vi "RDV-simpleGUI.vi"() -> ()   [LabVIEW 2020, in "RDV-Reflection_Data_viewer.lvclass"]
uses:
  RDV-Reflection_Data_viewer.lvclass
  RDV-PRELAUNCH_DATA.ctl
  RDV-XY_GRAPH_REFS.ctl
  RDV-GUI_REFS.ctl
panel:
  in  "Toggle Plot":bool
  in  "Stop":bool
  out "error out":errorcluster
  out "Permittivity Imag":T1(graph)
  out "Permittivity Real":T1(graph)
  out "Reflection Imag":T1(graph)
  out "Reflection Real":T1(graph)
  in  "Folder Path":path=path "C:/projects/Universitet/Master/data/Real Test - First libreVNA test with calibration file/Converted Data"
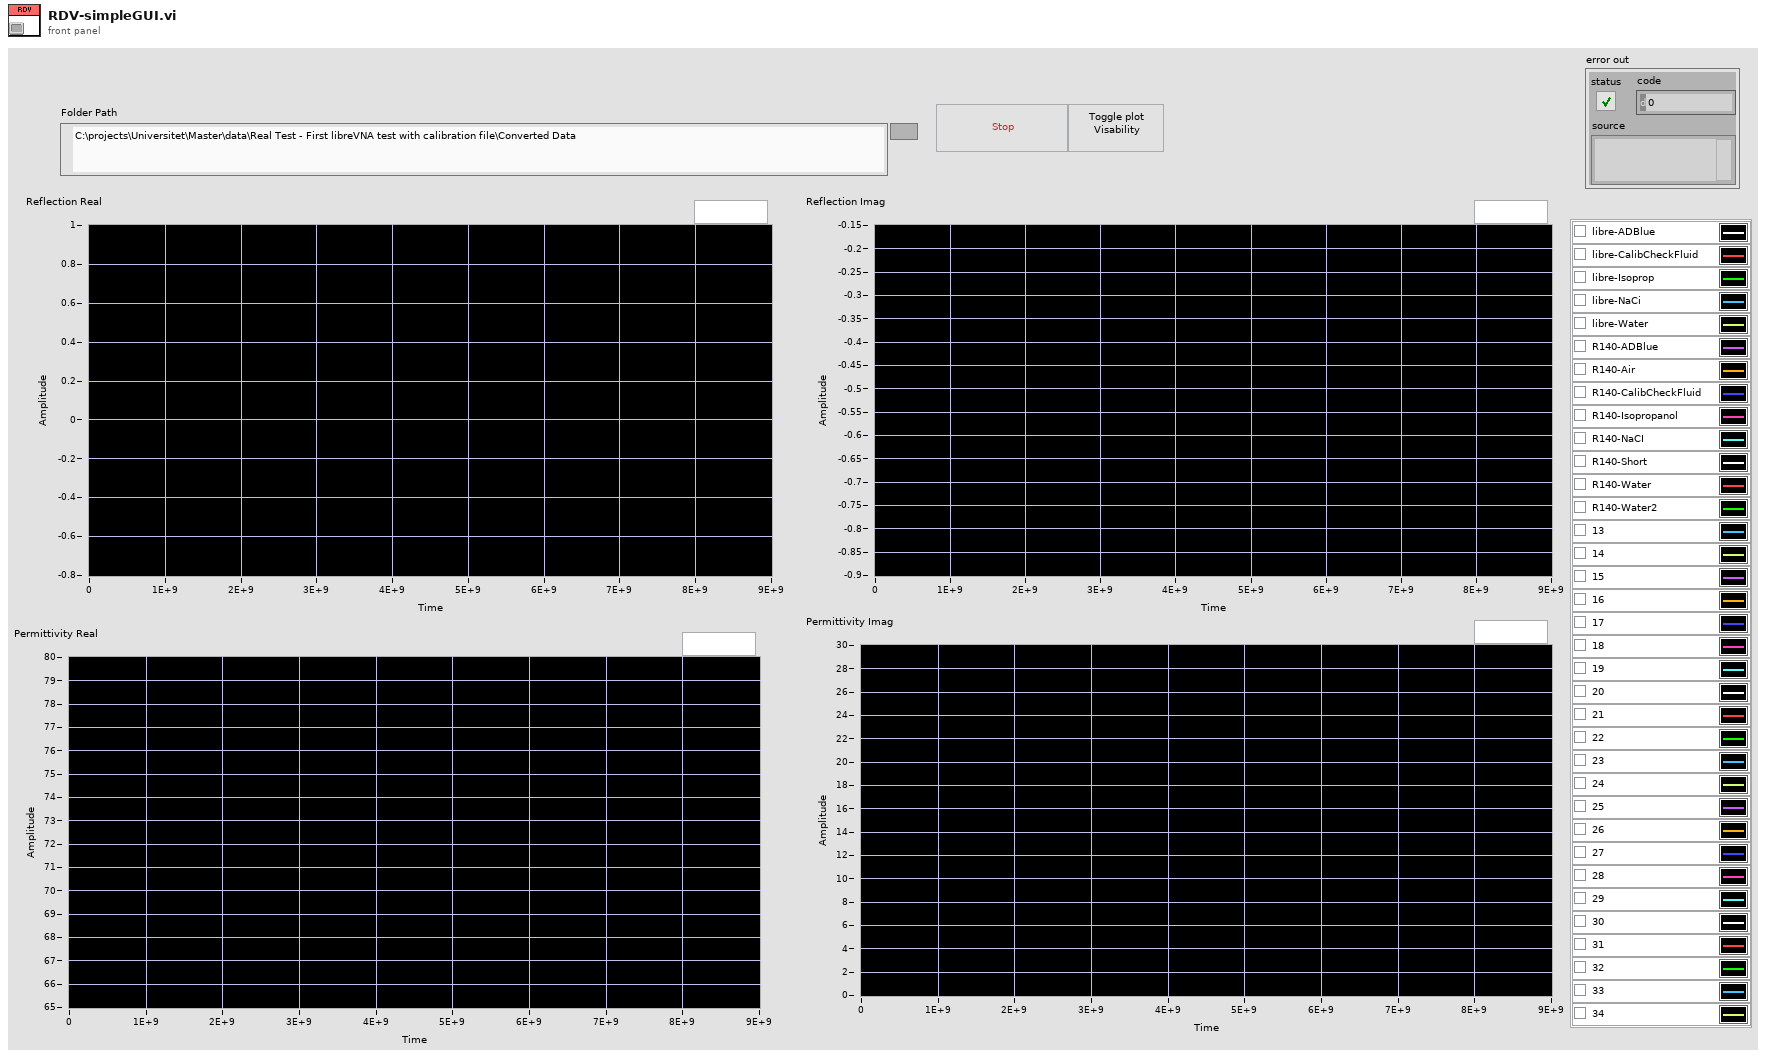
[diagram p1: front panel]
types:
  T1 = cluster{"Frequency":dbl[], "Reflection'":dbl[]}[]
  T2 = typedef "RDV-Reflection_Data_viewer.lvclass/RDV-PRELAUNCH_DATA.ctl" = cluster{"XY graph refs":T3, "GUI Refs":T4}
  T3 = typedef "RDV-Reflection_Data_viewer.lvclass/RDV-XY_GRAPH_REFS.ctl" = cluster{"Reflection Real":refnum<vi>, "Reflection Imag":refnum<vi>, "Permittivity Real":refnum<vi>, "Permittivity Imag":refnum<vi>}
  T4 = typedef "RDV-Reflection_Data_viewer.lvclass/RDV-GUI_REFS.ctl" = cluster{"Autoscale":refnum<vi>, "plot Selector":refnum<vi>[]}
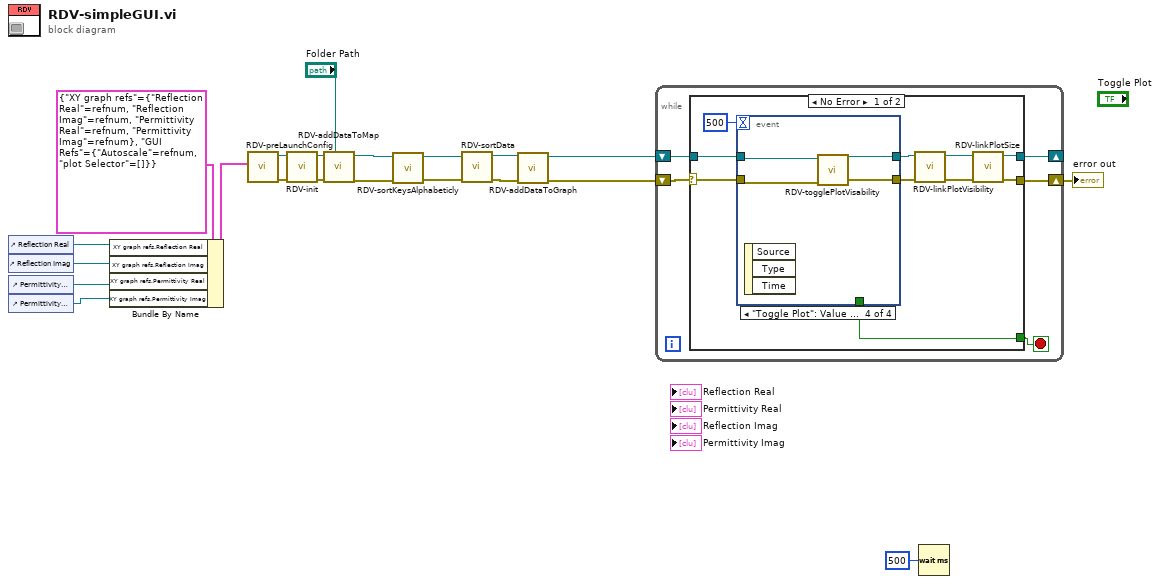
[diagram p0: block diagram]
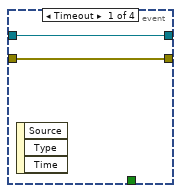
[diagram p2: hidden frame]
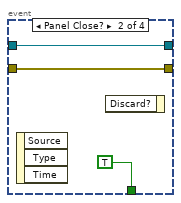
[diagram p3: hidden frame]
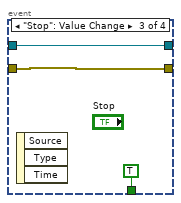
[diagram p4: hidden frame]
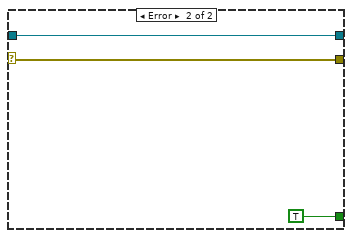
[diagram p5: hidden frame]
diagram:
  n1 = control-ref of="Reflection Real"() -> (w17:refnum<vi>)
  n2 = control-ref of="Reflection Imag"() -> (w16:refnum<vi>)
  n3 = control-ref of="Permittivity Real"() -> (w15:refnum<vi>)
  n4 = control-ref of="Permittivity Imag"() -> (w14:refnum<vi>)
  n5 = Bundle By Name(cluster=T2 {"XY graph refs"={"Reflection Real"=refnum, "Reflection Imag"=refnum, "Permittivity Real"=refnum, "Permittivity Imag"=refnum}, "GUI Refs"={"Autoscale"=refnum, "plot Selector"=[]}} ("preLaunch Config"), "XY graph refs.Reflection Real"=w17, "XY graph refs.Reflection Imag"=w16, "XY graph refs.Permittivity Real"=w15, "XY graph refs.Permittivity Imag"=w14) -> (w6:T2)
  n6 = call "RDV-preLaunchConfig.vi"("preLaunch Config"=w6) -> ("error out"=w2:errorcluster, "RDV-Reflection_Data_viewer out"=w3:refnum<class "RDV-Reflection_Data_viewer.lvclass">)  [unwired: 9 in]
  n7 = call "RDV-init.vi"("error in (no error)"=w2, "RDV-Reflection_Data_viewer in"=w3) -> ("error out"=w4:errorcluster, "RDV-Reflection_Data_viewer out"=w5:refnum<class "RDV-Reflection_Data_viewer.lvclass">)  [unwired: 8 in]
  n8 = call "RDV-addDataToMap.vi"("Folder Path"="Folder Path", "error in (no error)"=w4, "RDV-Reflection_Data_viewer in"=w5) -> ("error out"=w8:errorcluster, "RDV-Reflection_Data_viewer out"=w20:refnum<class "RDV-Reflection_Data_viewer.lvclass">)  [unwired: 7 in]
  n9 = call "RDV-sortKeysAlphabeticly.vi"("error in (no error)"=w8, "RDV-Reflection_Data_viewer in"=w20) -> ("error out"=w9:errorcluster, "RDV-Reflection_Data_viewer out"=w19:refnum<class "RDV-Reflection_Data_viewer.lvclass">)  [unwired: 8 in]
  n10 = call "RDV-sortData.vi"("error in (no error)"=w9, "RDV-Reflection_Data_viewer in"=w19) -> ("error out"=w10:errorcluster, "RDV-Reflection_Data_viewer out"=w13:refnum<class "RDV-Reflection_Data_viewer.lvclass">)  [unwired: 8 in]
  n11 = call "RDV-addDataToGraph.vi"("error in (no error)"=w10, "RDV-Reflection_Data_viewer in"=w13) -> ("error out"=w11:errorcluster, "RDV-Reflection_Data_viewer out"=w12:refnum<class "RDV-Reflection_Data_viewer.lvclass">)  [unwired: 8 in]
  n12 = while {
    shift-right: [w25] -> _
    shift-left: w12 -> [w26]
    shift-right: [w23] -> w7
    shift-left: w11 -> [w24]
    stop <- w22 stop-if-true
    n13 = case shown="No Error" w24 {
      selector: w24 -> [w29 w50]
      tunnel: w26 -> [w31 w51]
      tunnel: [w35 w51] -> w25
      tunnel: [w34 w50] -> w23
      tunnel: [w27 TRUE ("stop")] -> w22
      frame No Error {
        n14 = event shown="[3] \"Toggle Plot\": Value Change" {
          selector: _ -> [_ _ _ _]
          dyn-events: _ -> [_ _ _ _]
          timeout: 500 -> [_ _ _ _]
          tunnel: [w38 w40 w43 w48] -> w32
          tunnel: w31 -> [w38 w40 w43 w45]
          tunnel: [w37 w39 w42 w47] -> w30
          tunnel: w29 -> [w37 w39 w42 w46]
          tunnel: [_ TRUE ("Discard?") TRUE ("Discard?") _] -> w27
          event Timeout {
            n15 = event-data() -> ()  [unwired: 1 in, 3 out]
          }
          event Panel Close? {
            n16 = event-data() -> ()  [unwired: 1 in, 3 out]
            n17 = event-data() -> ()  [unwired: 2 in, 1 out]
          }
          event "Stop": Value Change {
            n18 = event-data() -> ()  [unwired: 1 in, 3 out]
          }
          event "Toggle Plot": Value Change {
            n19 = event-data() -> ()  [unwired: 1 in, 3 out]
            n20 = call "RDV-togglePlotVisability.vi"("error in (no error)"=w46, "RDV-Reflection_Data_viewer in"=w45) -> ("error out"=w47:errorcluster, "RDV-Reflection_Data_viewer out"=w48:refnum<class "RDV-Reflection_Data_viewer.lvclass">)  [unwired: 8 in]
          }
        }
        n21 = call "RDV-linkPlotVisibility.vi"("error in (no error)"=w30, "RDV-Reflection_Data_viewer in"=w32) -> ("error out"=w33:errorcluster, "RDV-Reflection_Data_viewer out"=w36:refnum<class "RDV-Reflection_Data_viewer.lvclass">)  [unwired: 8 in]
        n22 = call "RDV-linkPlotSize.vi"("error in (no error)"=w33, "RDV-Reflection_Data_viewer in"=w36) -> ("error out"=w34:errorcluster, "RDV-Reflection_Data_viewer out"=w35:refnum<class "RDV-Reflection_Data_viewer.lvclass">)  [unwired: 8 in]
      }
      frame Error {
      }
    }
  }
  "error out" <- w7
  n23 = Wait (ms)(milliseconds to wait=u32 500) -> ()  [unwired: 1 out]
